vi "Transmitter_Example.vi"() -> ()   [LabVIEW 2014]
uses:
  <instrlib>/niUSRP/niUSRP Write Tx Data (CDB Cluster).vi
panel:
  in  "Modulation parameter":T1
  out "Bits length":i32
  out "Frame Duration":dbl format="%#_6p"
  out "Waveform Graph":cluster{"t0":dbl, "dt":dbl, "Y":dbl[]}(graph)
  in  "stop":bool
  in  "String":string="如果采用顺序流接收的方式：先从USRP缓存区获取数据，分局数据确定物理层分组，再将分组传给下面的解调模块。由于解码耗时较长，会拖累获取数据的速度，使得从USRP缓存区获取数据的速率低于采样率，从而引发缓冲区爆满的问题。\n那么将接收和解调使用并行运行的方式：一个线程获取缓存区数据，并根据信号强度抽取出一个物理层分组，将分组放到共享队列里面；另一个线程监听该队列，一旦获取一个分组，就进行解调和解码。这种方式可以有效地解决缓存区爆满的问题。\n我真是太TM机制了"
  out "USRP CoercedParamters":T2={"coerced IQ rate"=100000.0, "coerced carrier frequency"=100000.0, "coerced gain"=0.0} {"coerced gain" format="%#_6f"; "coerced carrier frequency" format="%#_6p"; "coerced IQ rate" format="%#_6p"}
  out "error out":errorcluster
  in  "error in (no error)":errorcluster
  in  "USRP ControledParameters":T3={"active antenna"="TX1", "gain"=30.0, "carrier frequency"=5800000000.0, "IQ rate"=2000000.0} {"IQ rate" format="%#_6p"; "carrier frequency" format="%#_6p"; "gain" format="%#_6f"}
  in  "device names":refnum<k15>="NI2900"
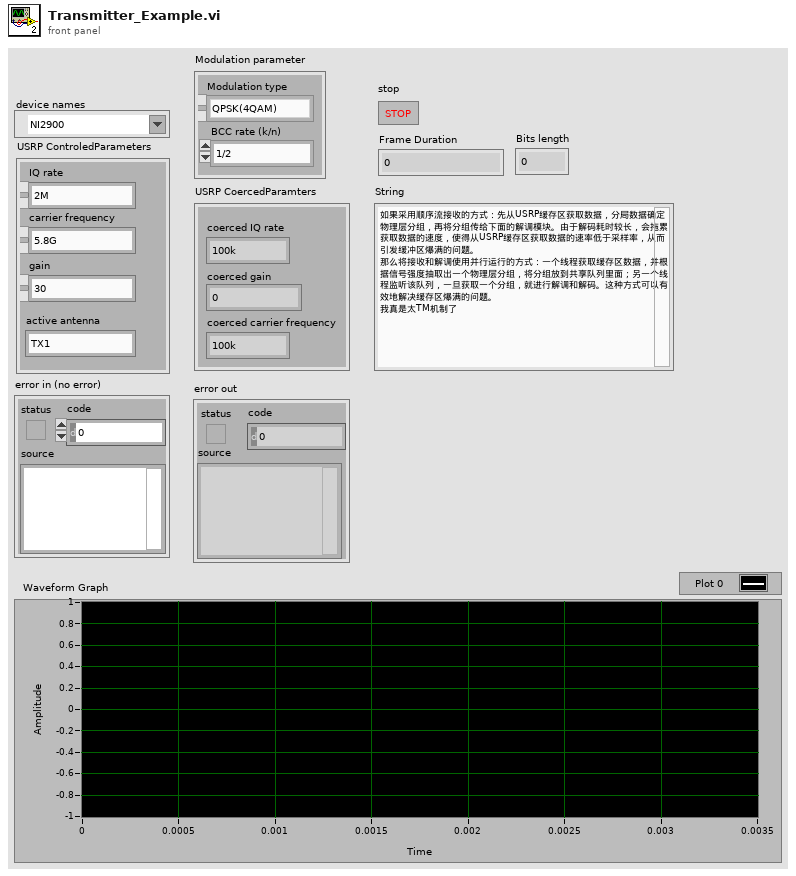
[diagram p1: front panel]
types:
  T1 = cluster{"Modulation type":enum16{"QPSK(4QAM)", "64QAM", "16QAM", "BPSK"}, "BCC rate (k/n)":enum16{"1/2", "2/3", "3/4"}}
  T2 = cluster{"coerced IQ rate":dbl, "coerced carrier frequency":dbl, "coerced gain":dbl}
  T3 = cluster{"active antenna":string, "gain":dbl, "carrier frequency":dbl, "IQ rate":dbl}
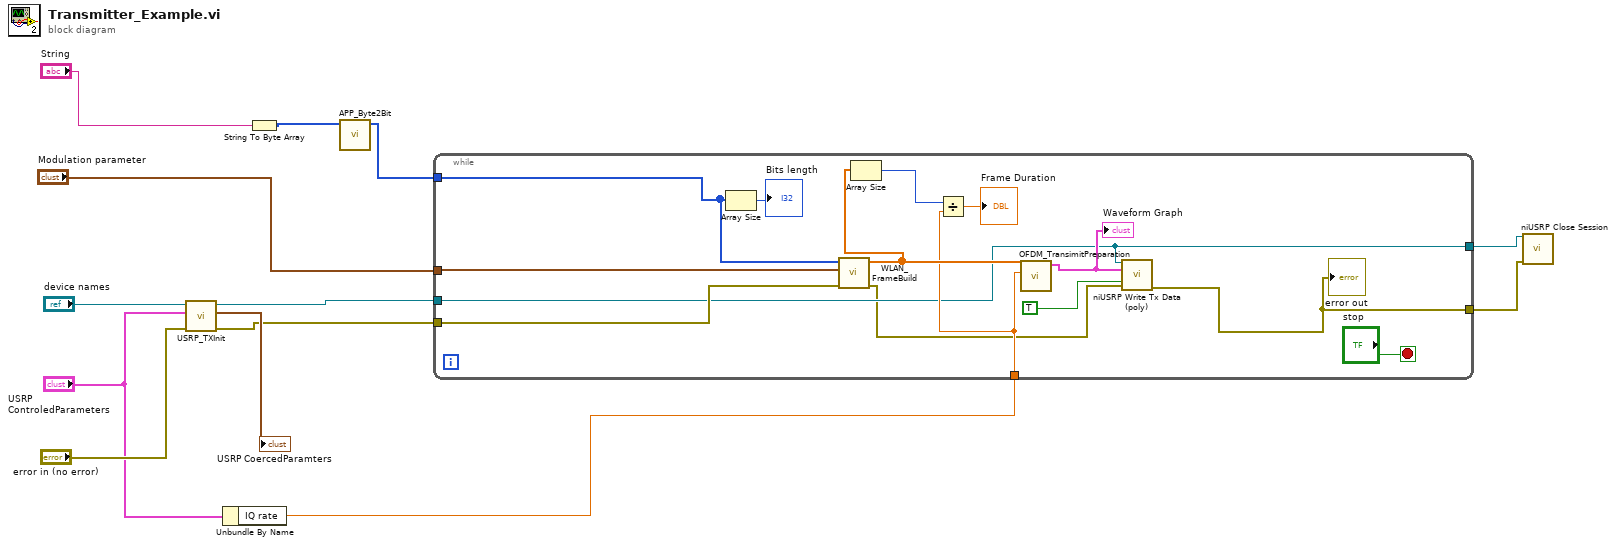
[diagram p0: block diagram]
diagram:
  n1 = call "USRP_TXInit.vi"("device names"="device names", "USRP ControledParameters"="USRP ControledParameters", "error in (no error)"="error in (no error)") -> ("session handle out"=w11:refnum<k15>, "USRP CoercedParamters"=→"USRP CoercedParamters":T2, "error out"=w7:errorcluster)  [unwired: 5 in]
  n2 = Unbundle By Name("USRP ControledParameters") -> ("IQ rate"=w6:dbl)
  n3 = String To Byte Array(string="String") -> (unsigned byte array=w2:u8[])
  n4 = call "APP_Byte2Bit.vi"("input byte stream"=w2) -> ("output bit stream"=w3:i8[])  [unwired: 10 in]
  n5 = while {
    tunnel: w11 -> [w17]
    tunnel: "Modulation parameter" -> [w25]
    tunnel: w7 -> [w24]
    tunnel: w6 -> [w20]
    tunnel: [w17] -> w5
    tunnel: [w16] -> w4
    tunnel: w3 -> [w14]
    stop <- "stop" stop-if-true
    n6 = Array Size(array=w14) -> (size(s)=→"Bits length":i32)
    n7 = call "WLAN_FrameBuild.vi"("error in (no error)"=w24, "Modulation parameter"=w25, "data in"=w14) -> ("error out"=w15:errorcluster, "output array"=w21:cdb[])  [unwired: 7 in]
    n8 = Array Size(array=w21) -> (size(s)=w23:i32)
    n9 = Divide(x=w23, y=w20) -> (x/y=→"Frame Duration":dbl)
    n10 = call "OFDM_TransimitPreparation.vi"("IQ rate"=w20, "array"=w21) -> ("output cluster"=w19:cluster{"t0":dbl, "dt":dbl, "Y":cdb[]})  [unwired: 9 in]
    "Waveform Graph" <- w19
    n11 = call-poly <instrlib>:"niUSRP Write Tx Data (poly).vi"("session handle"=w17, "data"=w19, "end of data?"=TRUE, "error in (no error)"=w15) -> ("error out"=w16:errorcluster)  [unwired: 10 in, 1 out]
    "error out" <- w16
  }
  n12 = call <instrlib>:"niUSRP Close Session.vi"("session handle"=w5, "error in (no error)"=w4) -> ()  [unwired: 13 in, 1 out]
